vi "Step Class Library FGV.vi"(8 "error in (no error)":errorcluster, 10 "Action":enum16{"Set", "Get"}(ring)=enum."Get", 11 "Step Type Class Library":T1) -> (0 "error out":errorcluster, 3 "Step Type Class Library out":T1)   [LabVIEW 2015, in "Configuration Tool.lvlib"]
uses:
  Configuration Tool.lvlib
  Controls/StepClassLibrary.ctl
  Prototype/classes/Step/Config/Step Config.lvclass
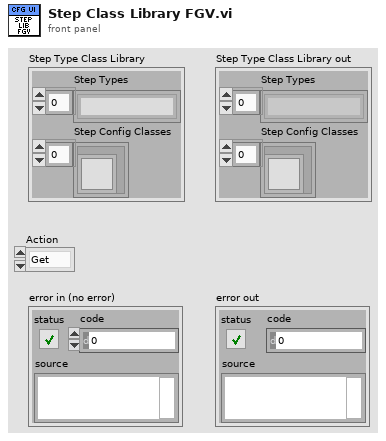
[diagram p1: front panel]
types:
  T1 = typedef "Configuration Tool.lvlib/StepClassLibrary.ctl" = cluster{"Step Types":string[], "Step Config Classes":refnum<class "Step Config.lvclass">[]}
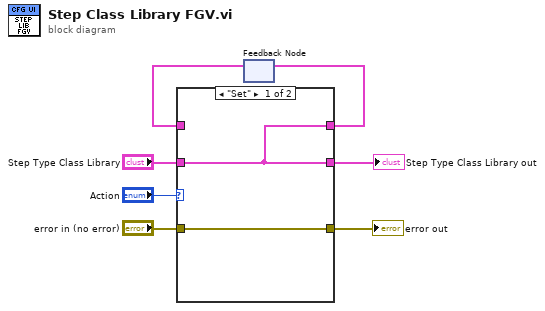
[diagram p0: block diagram]
diagram:
  n1 = feedback #1() -> (w1:T1)  [unwired: 1 in]
  n2 = case shown="\"Set\"" "Action" {
    tunnel: "Step Type Class Library" -> [w8 _]
    tunnel: [w8 w10] -> w6
    tunnel: "error in (no error)" -> [w9 w11]
    tunnel: [w9 w11] -> w4
    tunnel: [w8 w10] -> w2
    tunnel: w1 -> [_ w10]
    frame "Set" {
    }
    frame "Get", Default {
    }
  }
  "Step Type Class Library out" <- w6
  "error out" <- w4
  n3 = feedback-in #1(w2) -> ()
